vi "uni2(SubVI).vi"(6 "start":cluster{"x":dbl, "y":dbl}, 7 "goal":cluster{"x":dbl, "y":dbl}, 9 "xmax":dbl=1.0, 10 "xmin":dbl, 11 "dencity":i32=128) -> (3 "Array":cluster{"x":dbl, "y":dbl}[](array[cluster]))   [LabVIEW 2011]
uses:
  <vilib>/gmath/statdist.llb/Uniform Random.vi
  <vilib>/gmath/NI_Gmath.lvlib
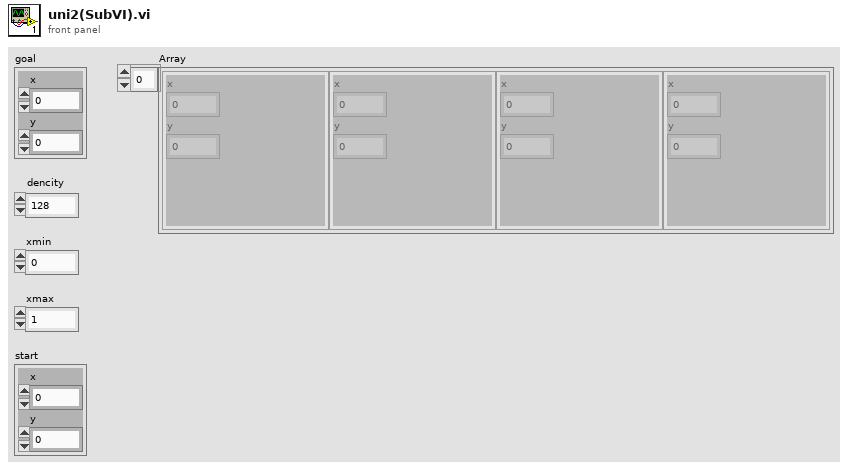
[diagram p1: front panel]
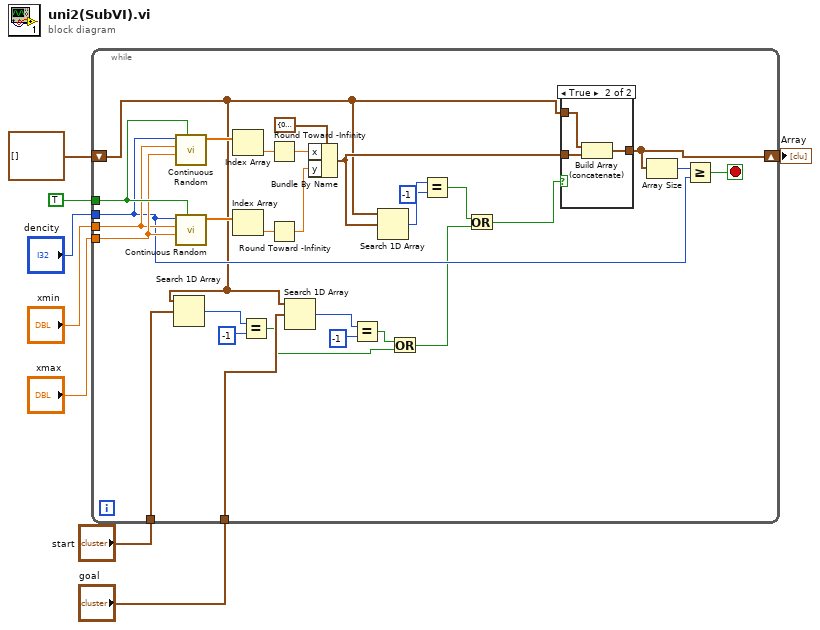
[diagram p0: block diagram]
diagram:
  n1 = while {
    tunnel: TRUE ("reset") -> [w37]
    tunnel: "xmax" -> [w36]
    tunnel: "xmin" -> [w35]
    tunnel: "dencity" -> [w22]
    shift-right: [w10] -> w3
    shift-left: cluster{"x":dbl, "y":dbl}[] [] -> [w9]
    tunnel: "start" -> [w21]
    tunnel: "goal" -> [w16]
    stop <- w23 stop-if-true
    n2 = Search 1D Array(1D array=w9, element=w21) -> (index of element=w19:i32)  [unwired: 1 in]
    n3 = call-poly <vilib>:"Continuous Random.vi"("reset"=w37, "xmax"=w36, "xmin"=w35, "samples"=w22) -> ("uniform random data"=w34:dbl[])  [unwired: 6 in, 1 out]
    n4 = call-poly <vilib>:"Continuous Random.vi"("reset"=w37, "xmax"=w36, "xmin"=w35, "samples"=w22) -> ("uniform random data"=w33:dbl[])  [unwired: 6 in, 1 out]
    n5 = Index Array(array=w34) -> (element=w32:dbl)  [unwired: 1 in]
    n6 = Index Array(array=w33) -> (element=w31:dbl)  [unwired: 1 in]
    n7 = Equal?(x=w19, y=-1) -> (x = y?=w14:bool)
    n8 = Round Toward -Infinity(1:w32) -> (0:w30:dbl)
    n9 = Round Toward -Infinity(1:w31) -> (0:w29:dbl)
    n10 = Search 1D Array(1D array=w9, element=w16) -> (index of element=w18:i32)  [unwired: 1 in]
    n11 = Bundle By Name(cluster=cluster{"x":dbl, "y":dbl} {"x"=0.0, "y"=0.0} ("input cluster"), "x"=w30, "y"=w29) -> (w25:cluster{"x":dbl, "y":dbl})
    n12 = Equal?(x=w18, y=-1) -> (x = y?=w15:bool)
    n13 = Search 1D Array(1D array=w9, element=w25) -> (index of element=w27:i32)  [unwired: 1 in]
    n14 = Or(x=w15, y=w14) -> (x .or. y?=w12:bool)
    n15 = Equal?(x=w27, y=-1) -> (x = y?=w13:bool)
    n16 = Or(x=w13, y=w12) -> (x .or. y?=w11:bool)
    n17 = case shown="True" w11 {
      tunnel: w25 -> [_ w41]
      tunnel: w9 -> [w38 w40]
      tunnel: [w38 w39] -> w10
      frame False {
      }
      frame True {
        n18 = Build Array (concatenate)(w40, w41) -> (w39:cluster{"x":dbl, "y":dbl}[])
      }
    }
    n19 = Array Size(array=w10) -> (size(s)=w24:i32)
    n20 = Greater Or Equal?(x=w24, y=w22) -> (x >= y?=w23:bool)
  }
  "Array" <- w3
